vi "Conversione csv.vi"(4 "Array 2":bool[][][](array[boolean]), 6 "Array di tabelle(usare build array) 2":string[][][](array[string]), 8 "Array":cluster{"index (row)":i32, "index (col)":i32}[](array[cluster]), 9 "Array tab risultati":string[][](array[string]), 11 "Array di tabelle(usare build array)":string[][][](array[string])) -> (3 "spreadsheet string":string)   [LabVIEW 2019]
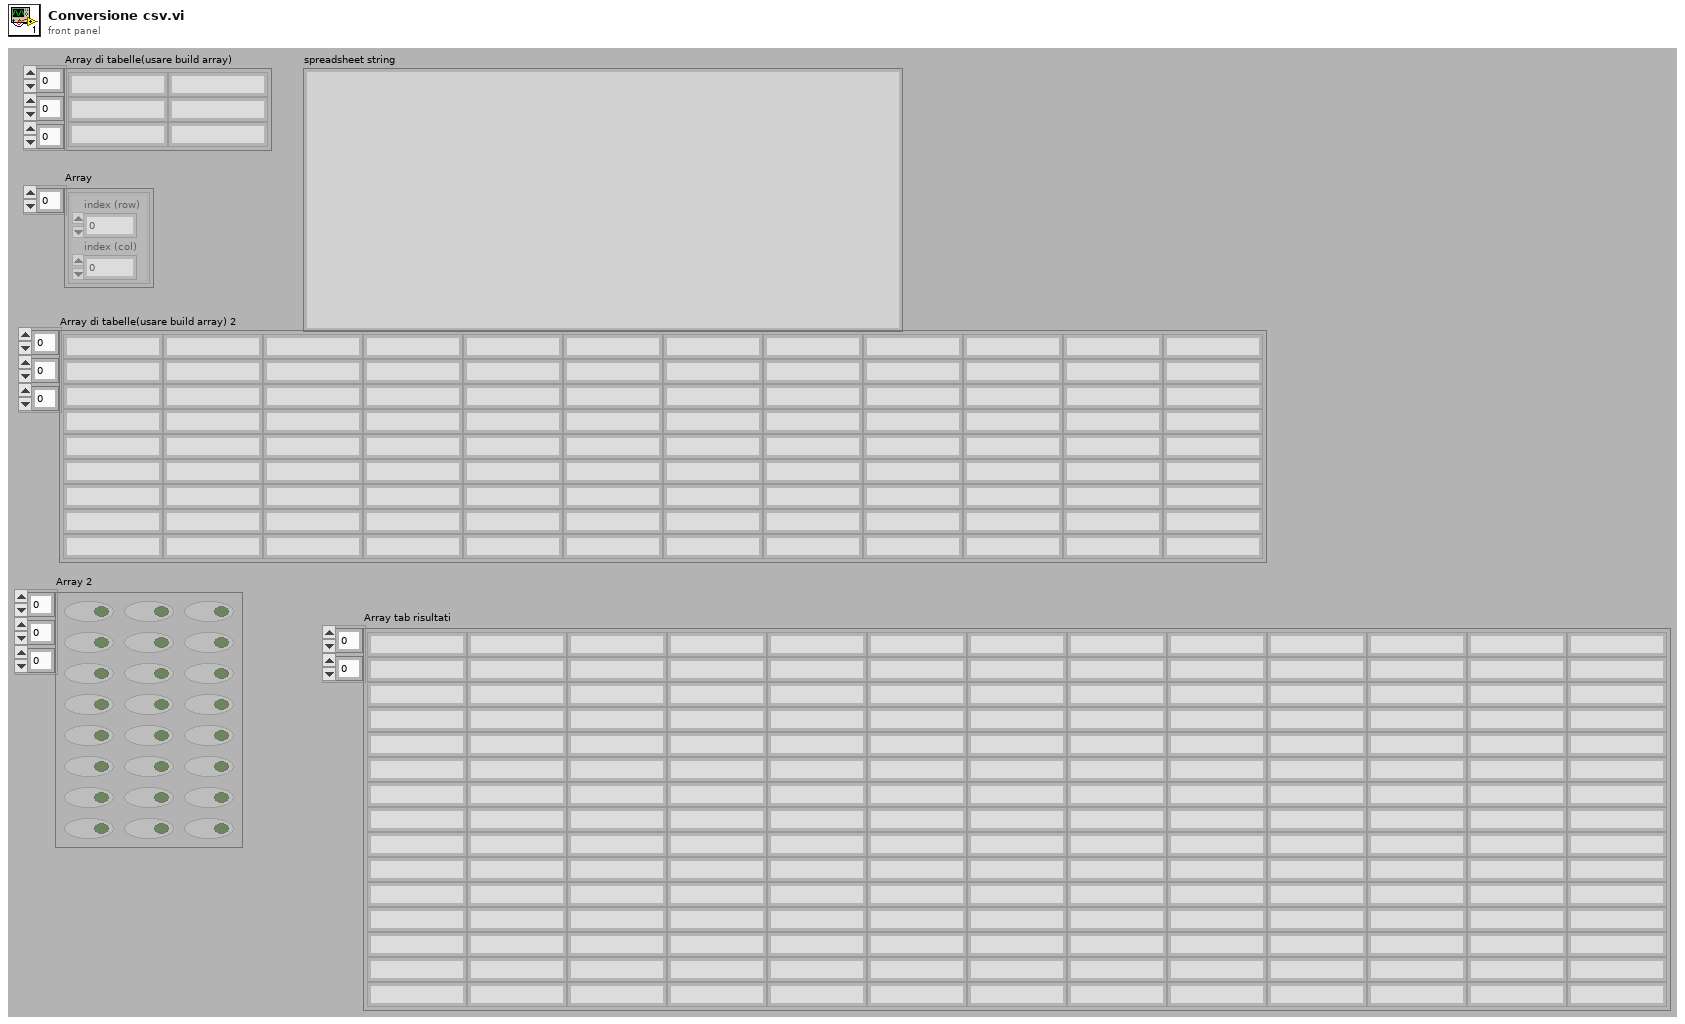
[diagram p1: front panel]
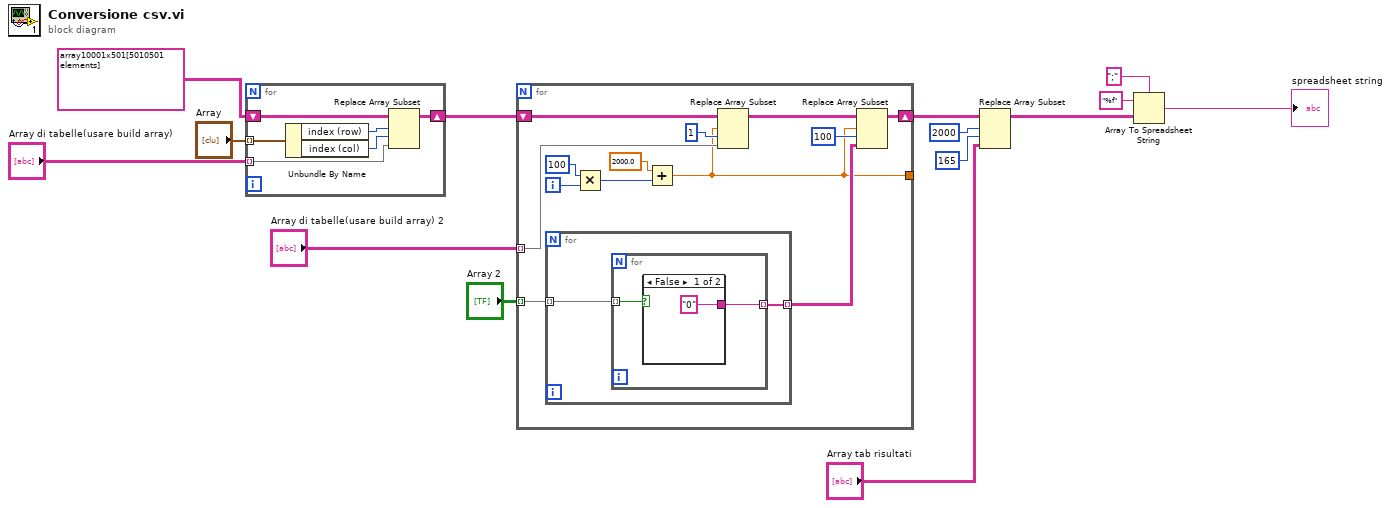
[diagram p0: block diagram]
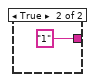
[diagram p2: hidden frame]
diagram:
  n1 = for {
    tunnel: "Array" -> [w20] mode=indexing
    tunnel: "Array di tabelle(usare build array)" -> [w17] mode=indexing
    shift-right: [w15] -> w6
    shift-left: string[][] array10001x501[5010501 elements] ("Array") -> [w16]
    n2 = Unbundle By Name(w20) -> ("index (row)"=w19:i32, "index (col)"=w18:i32)
    n3 = Replace Array Subset(array=w16, new element=w17, index (row)=w19, index (col)=w18) -> (w15:string[][])
  }
  n4 = for {
    tunnel: "Array di tabelle(usare build array) 2" -> [w33] mode=indexing
    shift-right: [w25] -> w5
    shift-left: w6 -> [w32]
    tunnel: "Array 2" -> [w23] mode=indexing
    tunnel: [w21] -> _
    i -> [w30]
    n5 = for {
      tunnel: w23 -> [w35] mode=indexing
      tunnel: [w34] -> w22 mode=indexing
      n6 = for {
        tunnel: w35 -> [w37] mode=indexing
        tunnel: [w36] -> w34 mode=indexing
        n7 = case shown="False" w37 {
          tunnel: ["0" "1"] -> w36
          frame False {
          }
          frame True {
          }
        }
      }
    }
    n8 = Multiply(x=100, y=w30) -> (x*y=w28:i32)
    n9 = Add(x=2000.0, y=w28) -> (x+y=w21:dbl)
    n10 = Replace Array Subset(array=w32, new element=w33, index (row)=w21, index (col)=1) -> (w26:string[][])
    n11 = Replace Array Subset(array=w26, new element=w22, index (row)=w21, index (col)=100 ("disabled index (col)")) -> (w25:string[][])
  }
  n12 = Replace Array Subset "Replace Array Subset"(array=w5, new element="Array tab risultati", index (row)=2000 ("disabled index (col)"), index (col)=165 ("disabled index (row)")) -> (w4:string[][])
  n13 = Array To Spreadsheet String(delimiter (Tab)=";", array=w4, 3:"%f") -> (spreadsheet string=→"spreadsheet string":string)
